vi "Configure Record Parameters.vi"   [LabVIEW 2011]
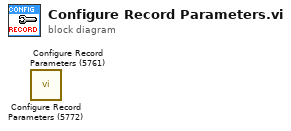
[diagram p0: block diagram]
diagram:
  n1 = call <userlib>:"Configure Record Parameters (5772).vi"() -> ()  [unwired: 9 in, 3 out]
  n2 = call <userlib>:"Configure Record Parameters (5761).vi"() -> ()  [unwired: 10 in, 2 out]
